vi "Stereo - Corresponding Points Dialog.vi"(10 "Right Image in":T1, 11 "Left Image in":T1) -> (2 "Right Image out":T1, 3 "Left Image out":T1)   [LabVIEW 2017]
doc: "Lets the user specify corresponding points on the left and right images."
uses:
  <vilib>/vision/Image Controls.llb/IMAQ Image.ctl
  <vilib>/vision/NI_Vision_Development_Module.lvlib
panel:
  out "error out":errorcluster
  in  "error in (no error)":errorcluster
  in  "OK":bool
  out "Right Image Point":T2 {"Calibration Quality" format="%#.5g"; "Max Distance" format="%#.4g"}
  out "Left Image Point":T2 {"Calibration Quality" format="%#.5g"; "Max Distance" format="%#.4g"}
  in  "Right Image":T1(plugin-control)
  in  "Left Image":T1(plugin-control)
  # "Click on the top left dot of the grid in each image"
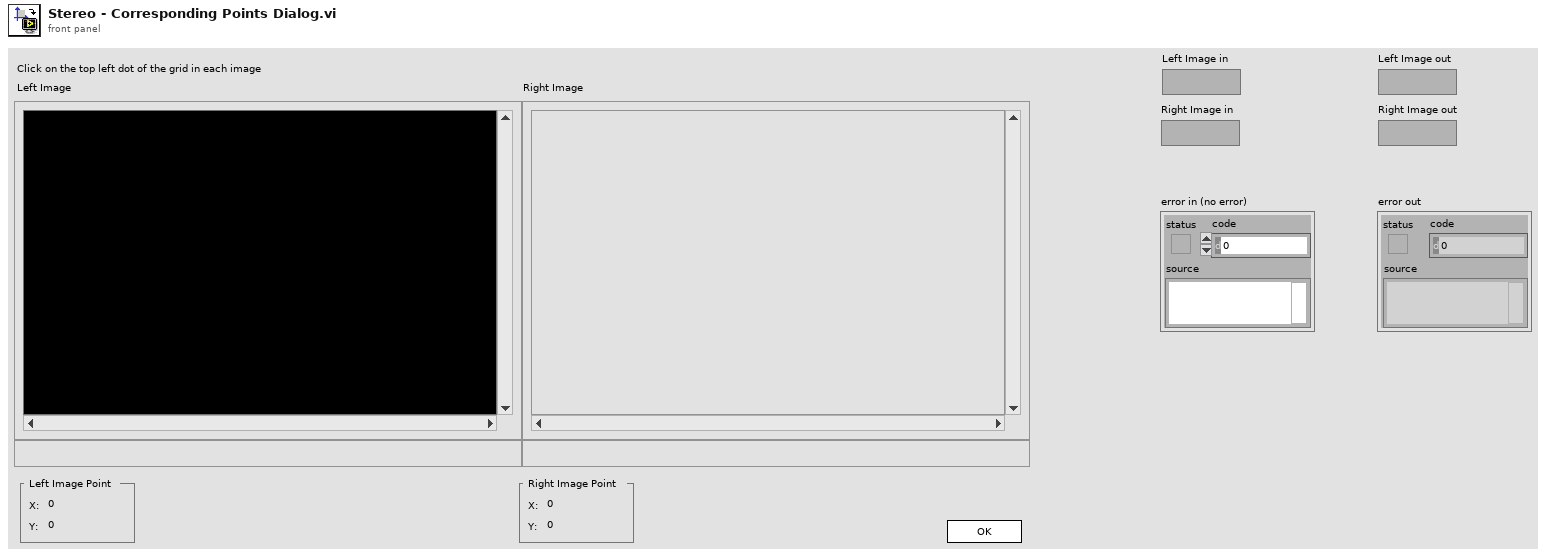
[diagram p1: front panel]
types:
  T1 = typedef "IMAQ Image.ctl" = refnum<image>
  T2 = cluster{"Max Distance":dbl, "Calibration Quality":dbl}
  T3 = cluster{"Origin Pixel":cluster{"X":sgl, "Y":sgl}, "Angle Relative to Horizontal (deg)":sgl, "Axis Reference":u32}
  T4 = cluster{"Max Distance":dbl, "Calibration Quality":dbl}[]
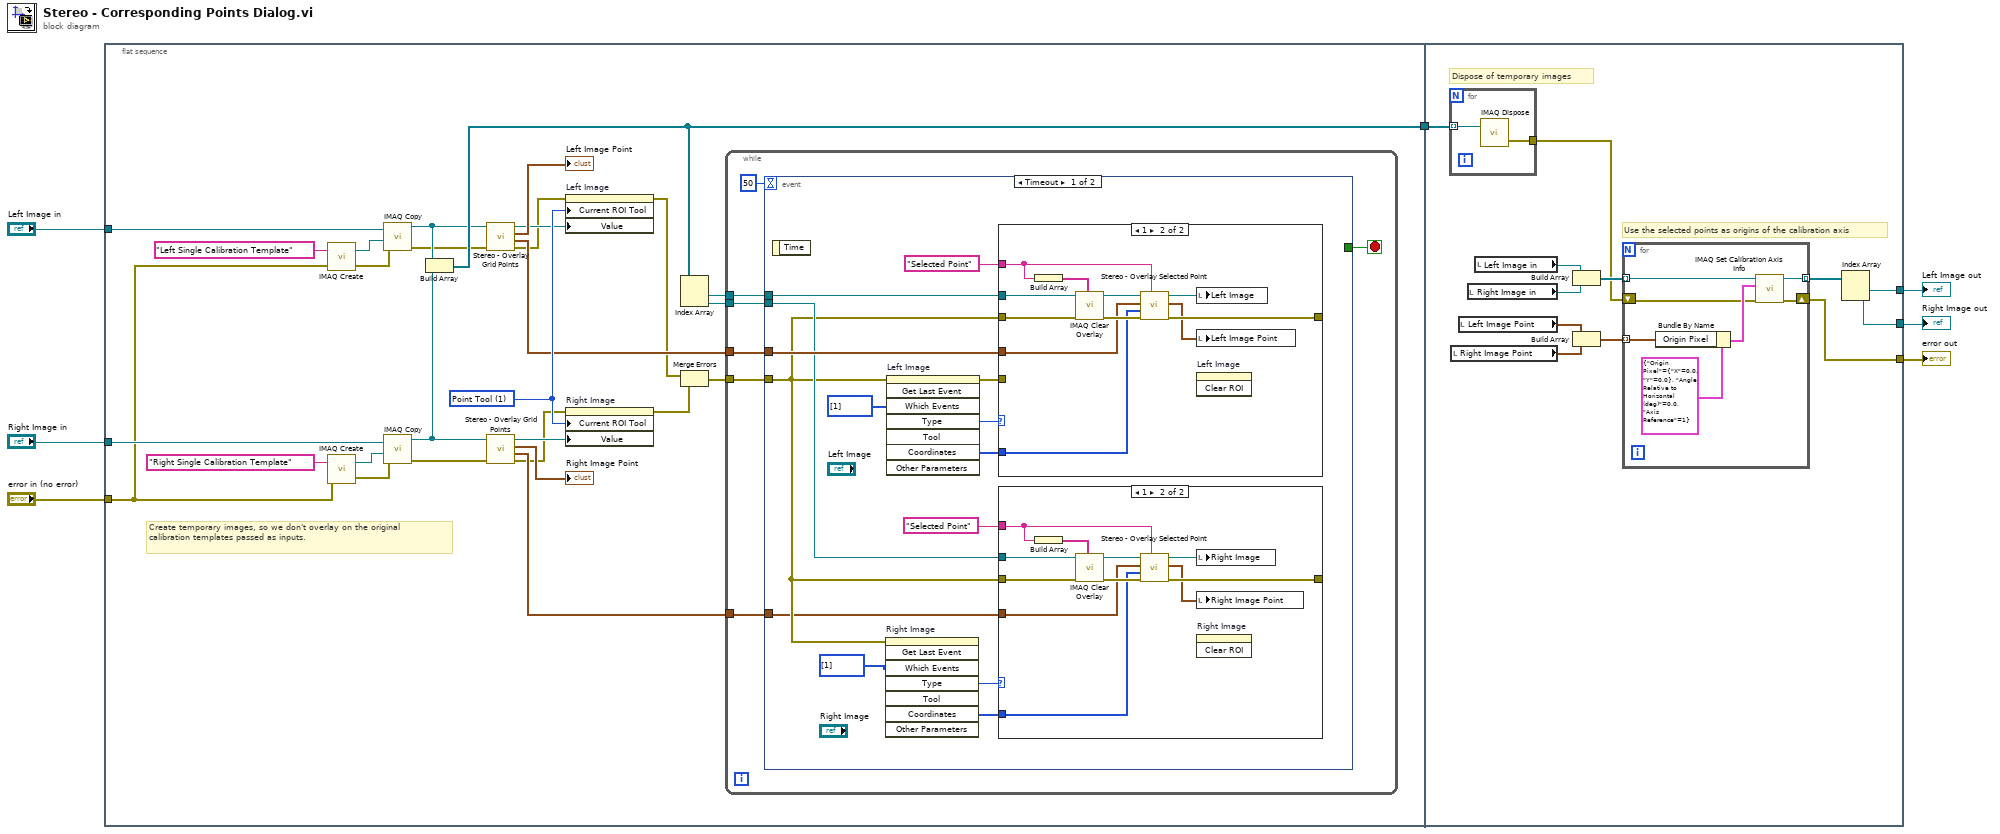
[diagram p0: block diagram]
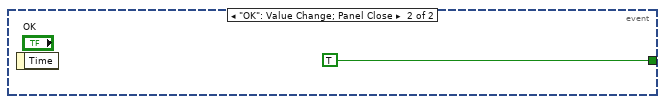
[diagram p4: hidden frame]
diagram:
  n1 = flat-sequence {
    tunnel: [w35] -> w3
    tunnel: "Left Image in" -> [w32]
    tunnel: "Right Image in" -> [w31]
    tunnel: "error in (no error)" -> [w17]
    tunnel: [w90] -> w5
    tunnel: [w89] -> w4
    tunnel: w3 -> [w91]
    tunnel: [w81] -> w1
    frame #0 {
      w30 = u32 1 items=["Zoom Tool"=8, "Selection Tool"=0, "Pan Tool"=9, "Point Tool"=1, "Line Tool"=2, "Rectangle Tool"=3, "Rotated Rectangle Tool"=12, "Polyline Tool"=10, "Polygon Tool"=5, "Freehand Tool"=11, "Closed Freehand Tool"=6, "Ellipse Tool"=4, "Annulus Tool"=7] ("Current ROI Tool")
      # "Create temporary images, so we don't overlay on the original calibration templates passed as inputs."
      n2 = call "IMAQ Create"("Image Name"="Left Single Calibration Template", "error in (no error)"=w17) -> ("New Image"=w27:T1, "error out"=w16:errorcluster)  [unwired: 2 in, 1 out]
      n3 = call "IMAQ Create"("Image Name"="Right Single Calibration Template", "error in (no error)"=w17) -> ("New Image"=w26:T1, "error out"=w15:errorcluster)  [unwired: 2 in, 1 out]
      n4 = call "IMAQ Copy"("error in (no error)"=w16, "Image Dst"=w27, "Image Src"=w32) -> ("error out"=w13:errorcluster, "Image Dst Out"=w19:T1)  [unwired: 3 out]
      n5 = call "IMAQ Copy"("error in (no error)"=w15, "Image Dst"=w26, "Image Src"=w31) -> ("error out"=w14:errorcluster, "Image Dst Out"=w18:T1)  [unwired: 3 out]
      n6 = Build Array(w19, w18) -> (w35:T1[])
      n7 = call "Stereo - Overlay Grid Points.vi"("error in (no error)"=w13, "Image in"=w19) -> ("error out"=w12:errorcluster, "Pixel Coordinates"=w23:cluster{"X":dbl, "Y":dbl}[], "Origin Pixel"=→"Left Image Point":cluster{"X":dbl, "Y":dbl}, "Image out"=w24:T1)  [unwired: 6 in]
      n8 = call "Stereo - Overlay Grid Points.vi"("error in (no error)"=w14, "Image in"=w18) -> ("error out"=w11:errorcluster, "Pixel Coordinates"=w22:cluster{"X":dbl, "Y":dbl}[], "Origin Pixel"=→"Right Image Point":cluster{"X":dbl, "Y":dbl}, "Image out"=w20:T1)  [unwired: 6 in]
      n9 = property on="Left Image" class="ImageControl"(error in=w12, "Current ROI Tool"=w30, "Value"=w24) -> (error out=w10:errorcluster)  [unwired: 1 in, 1 out]
      n10 = property on="Right Image" class="ImageControl"(error in=w11, "Current ROI Tool"=w30, "Value"=w20) -> (error out=w9:errorcluster)  [unwired: 1 in, 1 out]
      n11 = Index Array(array=w35) -> (element #1=w34:T1, element #2=w33:T1)  [unwired: 2 in]
      n12 = Merge Errors(w10, w9) -> (w8:errorcluster)
      n13 = while {
        tunnel: w23 -> [w40]
        tunnel: w34 -> [w39]
        tunnel: w22 -> [w38]
        tunnel: w33 -> [w37]
        tunnel: w8 -> [w36]
        stop <- w42 stop-if-true
        n14 = event shown="[0] Timeout" {
          selector: _ -> [_ _]
          dyn-events: _ -> [_ _]
          timeout: 50 -> [_ _]
          tunnel: [_ TRUE] -> w42
          tunnel: w40 -> [w56 _]
          tunnel: w39 -> [w55 _]
          tunnel: w38 -> [w45 _]
          tunnel: w37 -> [w47 _]
          tunnel: w36 -> [w46 _]
          event Timeout {
            n15 = event-data() -> ()  [unwired: 2 out]
            n16 = invoke on="Right Image" class="ImageControl" method="Get Last Event"(error in=w46, "Which Events"=i32[] [1]) -> ("Type"=w44:i32, "Coordinates"=w43:i32[])  [unwired: 6 in, 6 out]
            n17 = invoke on="Left Image" class="ImageControl" method="Get Last Event"(error in=w46, "Which Events"=i32[] [1]) -> (error out=w49:errorcluster, "Type"=w52:i32, "Coordinates"=w51:i32[])  [unwired: 6 in, 5 out]
            n18 = case shown="1" w52 {
              tunnel: w51 -> [_ w70]
              tunnel: w56 -> [_ w71]
              tunnel: w55 -> [_ w77]
              tunnel: "Selected Point" ("String") -> [_ w68]
              tunnel: w49 -> [_ _]
              tunnel: w46 -> [_ w76]
              tunnel: [_ w72] -> _
              frame 0, Default {
              }
              frame 1 {
                n19 = Build Array(w68) -> (w78:string[])
                n20 = call "IMAQ Clear Overlay"("Groups"=w78, "error in (no error)"=w76, "Image"=w77) -> ("error out"=w73:errorcluster, "Image Out"=w75:T1)  [unwired: 7 out]
                n21 = call "Stereo - Overlay Selected Point.vi"("Group"=w68, "error in (no error)"=w73, "Point Coordinates"=w70, "Points"=w71, "Image in"=w75) -> ("error out"=w72:errorcluster, "Point out"=w69:cluster{"X":dbl, "Y":dbl}, "Image out"=w74:T1)  [unwired: 4 in]
                n22 = local write "Left Image"(w74) -> ()
                n23 = local write "Left Image Point"(w69) -> ()
                n24 = invoke on="Left Image" class="ImageControl" method="Clear ROI"() -> ()  [unwired: 3 in, 3 out]
              }
            }
            n25 = case shown="1" w44 {
              tunnel: w43 -> [_ w59]
              tunnel: w45 -> [_ w60]
              tunnel: w47 -> [_ w66]
              tunnel: "Selected Point" ("String") -> [_ w57]
              tunnel: w46 -> [_ w65]
              tunnel: [_ w61] -> _
              frame 0, Default {
              }
              frame 1 {
                n26 = Build Array(w57) -> (w67:string[])
                n27 = call "IMAQ Clear Overlay"("Groups"=w67, "error in (no error)"=w65, "Image"=w66) -> ("error out"=w62:errorcluster, "Image Out"=w64:T1)  [unwired: 7 out]
                n28 = call "Stereo - Overlay Selected Point.vi"("Group"=w57, "error in (no error)"=w62, "Point Coordinates"=w59, "Points"=w60, "Image in"=w64) -> ("error out"=w61:errorcluster, "Point out"=w58:cluster{"X":dbl, "Y":dbl}, "Image out"=w63:T1)  [unwired: 4 in]
                n29 = local write "Right Image"(w63) -> ()
                n30 = local write "Right Image Point"(w58) -> ()
                n31 = invoke on="Right Image" class="ImageControl" method="Clear ROI"() -> ()  [unwired: 3 in, 3 out]
              }
            }
          }
          event "OK": Value Change; Panel Close {
            n32 = event-data() -> ()  [unwired: 2 out]
          }
        }
      }
    }
    frame #1 {
      # "Use the selected points as origins of the calibration axis"
      # "Dispose of temporary images"
      n33 = for {
        tunnel: w91 -> [w100] mode=indexing
        tunnel: [w99] -> w80
        n34 = call "IMAQ Dispose"("Image"=w100) -> ("error out"=w99:errorcluster)  [unwired: 2 in, 3 out]
      }
      n35 = local read "Right Image Point"() -> (w87:T2)
      n36 = local read "Left Image Point"() -> (w88:T2)
      n37 = local read "Right Image in"() -> (w82:T1)
      n38 = local read "Left Image in"() -> (w83:T1)
      n39 = Build Array(w83, w82) -> (w84:T1[])
      n40 = Build Array(w88, w87) -> (w86:T4)
      n41 = for {
        tunnel: w84 -> [w98] mode=indexing
        tunnel: w86 -> [w96] mode=indexing
        tunnel: [w94] -> w85 mode=indexing
        shift-right: [w92] -> w81
        shift-left: w80 -> [w93]
        n42 = Bundle By Name(cluster=T3 {"Origin Pixel"={"X"=0.0, "Y"=0.0}, "Angle Relative to Horizontal (deg)"=0.0, "Axis Reference"=1} ("Calibration Axis Info"), "Origin Pixel"=w96) -> (w95:T3)
        n43 = call "IMAQ Set Calibration Axis Info"("error in (no error)"=w93, "Calibration Axis Info"=w95, "Calibration Template Image In"=w98) -> ("error out"=w92:errorcluster, "Calibration Template Image Out"=w94:T1)  [unwired: 7 out]
      }
      n44 = Index Array(array=w85) -> (element #1=w90:T1, element #2=w89:T1)  [unwired: 2 in]
    }
  }
  "Left Image out" <- w5
  "Right Image out" <- w4
  "error out" <- w1
